vi "recipeWriteToIndicator.vi"(10 "Value":i32, 11 "Item Names":string[](array[string])) -> (2 "Cluster":T1)   [LabVIEW 2021]
uses:
  <vilib>/Utility/xml.llb/Read From XML File(array).vi
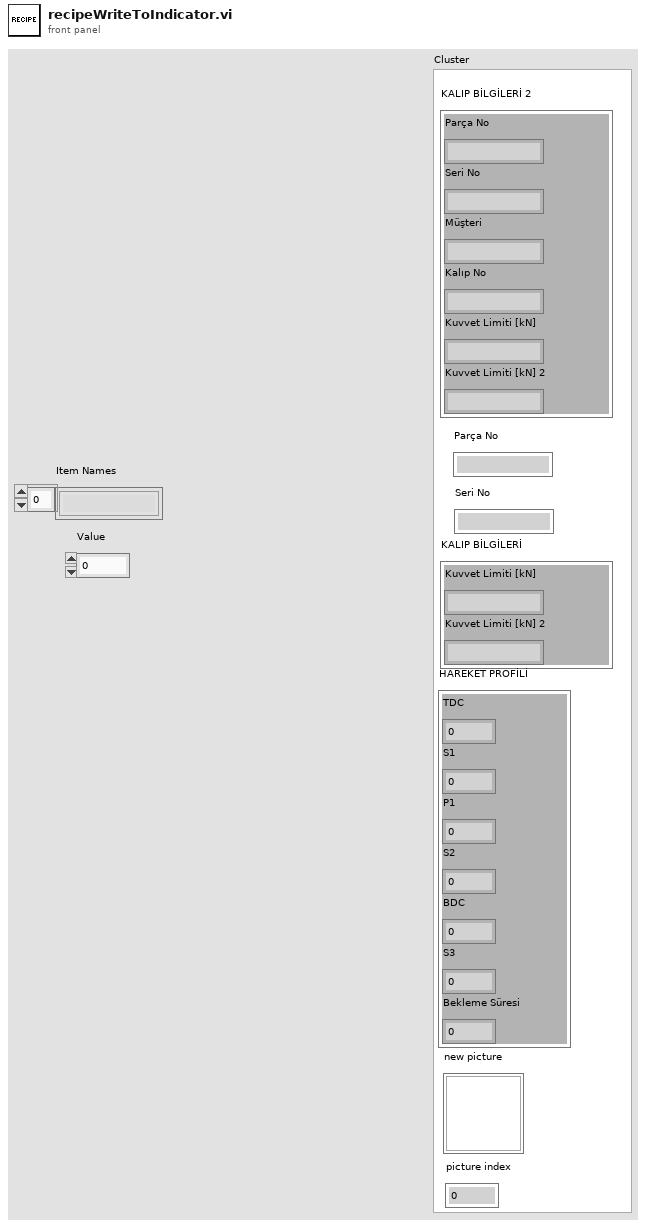
[diagram p1: front panel]
types:
  T1 = cluster{"KALIP BİLGİLERİ 2":cluster{"Parça No":string, "Seri No":string, "Müşteri":string, "Kalıp No":string, "Kuvvet Limiti [kN]":string, "Kuvvet Limiti [kN] 2":string}, "Parça No":string, "Seri No":string, "KALIP BİLGİLERİ":cluster{"Kuvvet Limiti [kN]":string, "Kuvvet Limiti [kN] 2":string}, "HAREKET PROFİLİ":cluster{"TDC":dbl, "S1":dbl, "P1":dbl, "S2":dbl, "BDC":dbl, "S3":dbl, "Bekleme Süresi":dbl}, "new picture":picture, "picture index":dbl}
  T2 = cluster{"Parça No":string, "Seri No":string, "Müşteri":string, "Kalıp No":string, "Kuvvet Limiti [kN]":string, "Kuvvet Limiti [kN] 2":string}
  T3 = cluster{"Kuvvet Limiti [kN]":string, "Kuvvet Limiti [kN] 2":string}
  T4 = cluster{"TDC":dbl, "S1":dbl, "P1":dbl, "S2":dbl, "BDC":dbl, "S3":dbl, "Bekleme Süresi":dbl}
  T5 = typedef "imagedata.ctl" = cluster{"image type":i32, "image depth":i32, "image":u8[], "mask":u8[], "colors":u32[], "Rectangle":cluster{"left":i16, "top":i16, "right":i16, "bottom":i16}}
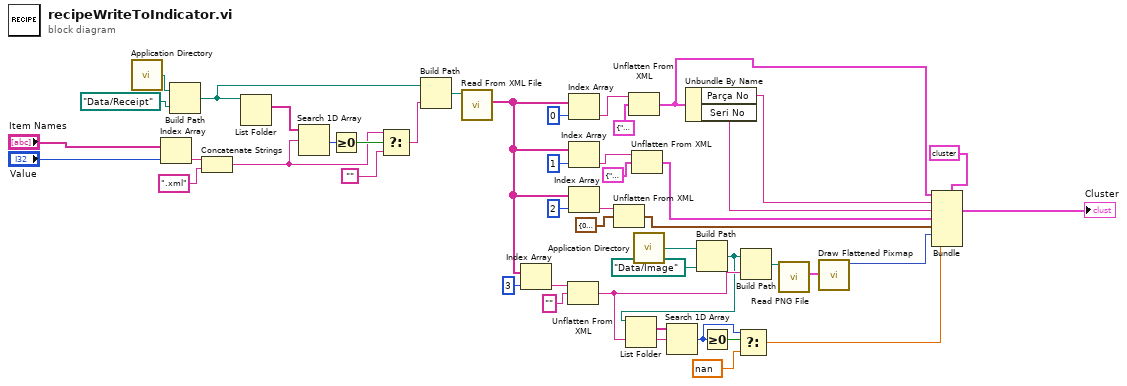
[diagram p0: block diagram]
diagram:
  n1 = call <vilib>:"Application Directory.vi"() -> ("Application Directory"=w20:path)
  n2 = Index Array(array="Item Names", index="Value") -> (element=w19:string)
  n3 = Build Path(base path=w20, name or relative path=path "Data/Receipt") -> (appended path=w14:path)
  n4 = Concatenate Strings(w19, ".xml") -> (w15:string)
  n5 = List Folder(path=w14) -> (filenames=w18:string[])  [unwired: 3 in, 3 out]
  n6 = Search 1D Array(1D array=w18, element=w15) -> (index of element=w17:i32)  [unwired: 1 in]
  n7 = Greater Or Equal To 0?(x=w17) -> (x >= 0?=w16:bool)
  n8 = Select(t=w15, s=w16, f="") -> (s? t:f=w12:string)
  n9 = Build Path(base path=w14, name or relative path=w12) -> (appended path=w13:path)
  n10 = call-poly <vilib>:"Read From XML File.vi"("XML File Path"=w13) -> ("XML Elements"=w35:string[])  [unwired: 8 in, 2 out]
  n11 = Index Array(array=w35, index=3) -> (element=w36:string)
  n12 = Unflatten From XML(xml string=w36, type="" ("anything")) -> (value=w43:string)  [unwired: 1 in, 1 out]
  n13 = Index Array(array=w35, index=0) -> (element=w25:string)
  n14 = Index Array(array=w35, index=1) -> (element=w31:string)
  n15 = Index Array(array=w35, index=2) -> (element=w24:string)
  n16 = Unflatten From XML(xml string=w24, type=T4 {"TDC"=0.0, "S1"=0.0, "P1"=0.0, "S2"=0.0, "BDC"=0.0, "S3"=0.0, "Bekleme Süresi"=0.0} ("HAREKET PROFİLİ")) -> (value=w3:T4)  [unwired: 1 in, 1 out]
  n17 = Unflatten From XML(xml string=w25, type=T2 {"Parça No"="111445", "Seri No"="565", "Müşteri"="Mercedes-Benz", "Kalıp No"="6666", "Kuvvet Limiti [kN]"="1000", "Kuvvet Limiti [kN] 2"="1000"} ("KALIP BİLGİLERİ")) -> (value=w7:T2)  [unwired: 1 in, 1 out]
  n18 = Unflatten From XML(xml string=w31, type=T3 {"Kuvvet Limiti [kN]"="", "Kuvvet Limiti [kN] 2"=""} ("KALIP BİLGİLERİ")) -> (value=w4:T3)  [unwired: 1 in, 1 out]
  n19 = call <vilib>:"Application Directory.vi"() -> ("Application Directory"=w37:path)
  n20 = Unbundle By Name(w7) -> ("Parça No"=w6:string, "Seri No"=w5:string)
  n21 = Build Path(base path=w37, name or relative path=path "Data/Image") -> (appended path=w41:path)
  n22 = List Folder(path=w41) -> (filenames=w42:string[])  [unwired: 3 in, 3 out]
  n23 = Search 1D Array(1D array=w42, element=w43) -> (index of element=w45:i32)  [unwired: 1 in]
  n24 = Greater Or Equal To 0?(x=w45) -> (x >= 0?=w44:bool)
  n25 = Select(t=w45, s=w44, f=nan) -> (s? t:f=w1:dbl)
  n26 = Build Path(base path=w41, name or relative path=w43) -> (appended path=w40:path)
  n27 = call <vilib>:"Read PNG File.vi"("path to PNG file"=w40) -> ("image data"=w39:T5)  [unwired: 8 in, 2 out]
  n28 = call <vilib>:"Draw Flattened Pixmap.vi"("image data"=w39) -> ("new picture"=w2:picture)  [unwired: 8 in]
  n29 = Bundle(cluster=T1 {"KALIP BİLGİLERİ 2"={"Parça No"="", "Seri No"="", "Müşteri"="", "Kalıp No"="", "Kuvvet Limiti [kN]"="", "Kuvvet Limiti [kN] 2"=""}, "Parça No"="", "Seri No"="", "KALIP BİLGİLERİ"={"Kuvvet Limiti [kN]"="", "Kuvvet Limiti [kN] 2"=""}, "HAREKET PROFİLİ"={"TDC"=0.0, "S1"=0.0, "P1"=0.0, "S2"=0.0, "BDC"=0.0, "S3"=0.0, "Bekleme Süresi"=0.0}, "new picture"=bytes[0], "picture index"=0.0} ("Cluster"), "KALIP BİLGİLERİ 2"=w7, "Parça No"=w6, "Seri No"=w5, "KALIP BİLGİLERİ"=w4, "HAREKET PROFİLİ"=w3, "new picture"=w2, "picture index"=w1) -> (→"Cluster":T1)
